vi "LAC Cmd121_ZOOM.vi"(6 "R/W (F:Read)":bool, 7 "timeout(ms)":u32, 8 "error in":errorcluster, 9 "zoom_val":T1, 11 "VISA name in":refnum<visa-resource-name>) -> (0 "error out":errorcluster, 1 "readout":string, 3 "VISA name out":refnum<visa-resource-name>)   [LabVIEW 8.6]
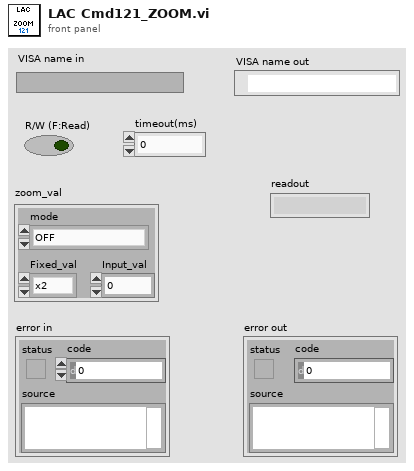
[diagram p1: front panel]
types:
  T1 = cluster{"mode":enum16{"OFF", "Fixed value", "Input value"}, "Fixed_val":enum16{"x2", "x4", "x8"}, "Input_val":dbl}
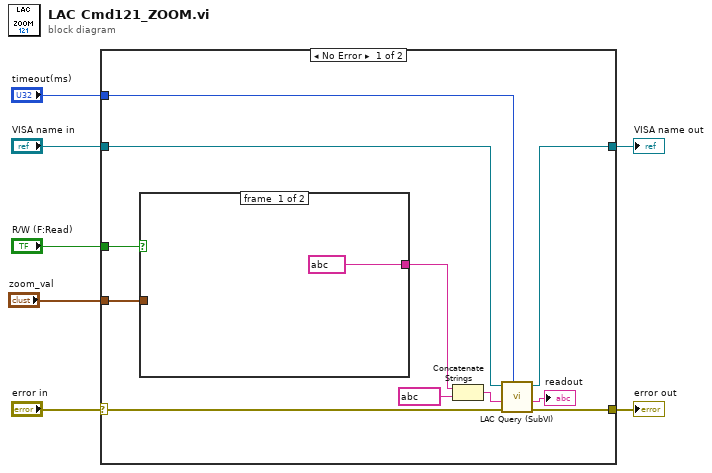
[diagram p0: block diagram]
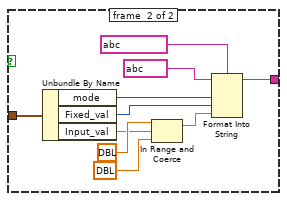
[diagram p2: hidden frame]
diagram:
  n1 = case shown="No Error" "error in" {
    selector: "error in" -> [w14 w31]
    tunnel: "VISA name in" -> [w16 w30]
    tunnel: [w18 w30] -> w6
    tunnel: [w17 w31] -> w5
    tunnel: "timeout(ms)" -> [w15 _]
    tunnel: "R/W (F:Read)" -> [w9 _]
    tunnel: "zoom_val" -> [w8 _]
    frame #0 {
      n2 = case shown="True" w9 {
        tunnel: [string ? ("string") w27] -> w10
        tunnel: w8 -> [_ w23]
        frame #0 {
        }
        frame #1 {
          n3 = Unbundle By Name(w23) -> ("mode"=w20:enum16{"OFF", "Fixed value", "Input value"}, "Fixed_val"=w21:enum16{"x2", "x4", "x8"}, "Input_val"=w22:dbl)
          n4 = In Range and Coerce(upper limit=dbl ?, x=w22, lower limit=dbl ?) -> (coerced(x)=w26:dbl)  [unwired: 1 out]
          n5 = Format Into String(format string=string ?, initial string=string ? ("string"), w20, w21, w26) -> (resulting string=w27:string)  [unwired: 1 in, 1 out]
        }
      }
      n6 = Concatenate Strings(w10, string ? ("write buffer")) -> (w12:string)
      n7 = call "LAC Query (SubVI).vi"("timeout(ms)"=w15, "error in"=w14, "Command"=w12, "VISA name in"=w16) -> ("error out"=w17:errorcluster, "read buffer"=→"readout":string, "VISA name out"=w18:refnum<visa-resource-name>)  [unwired: 5 in]
    }
    frame #1 {
    }
  }
  "VISA name out" <- w6
  "error out" <- w5
